vi "Post Process Noise Filter.vi"(0 "pInputImage":i32, 1 "iMode":i32, 2 "iHeight":i32, 5 "pOutputImage":i32, 7 "iOutputBufferSize":i32, 9 "iBaseline":i32, 11 "error in (no error)":errorcluster, 12 "fThreshold":sgl, 13 "iWidth":i32) -> (4 "pInputImage out":i32, 6 "pOutputImage out":i32, 8 "function return":u32, 15 "error out":errorcluster)   [LabVIEW 2014, in "atmcd32d.lvlib"]
doc: "unsigned int WINAPI PostProcessNoiseFilter(at_32 * pInputImage, at_32 * pOutputImage, int iOutputBufferSize, int iBaseline, int iMode, float fThreshold, int iHeight, int iWidth);"
uses:
  atmcd32d.lvlib
  atmcd32d.dll
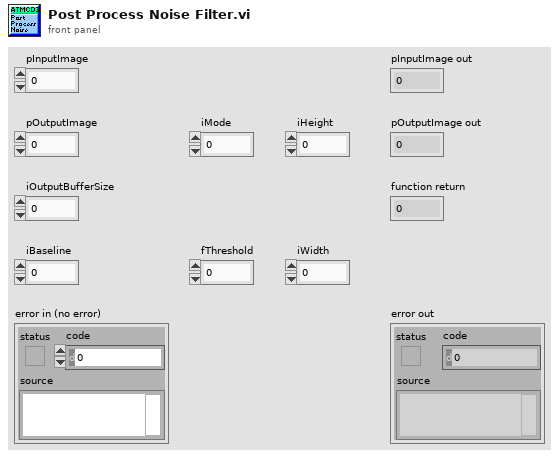
[diagram p1: front panel]
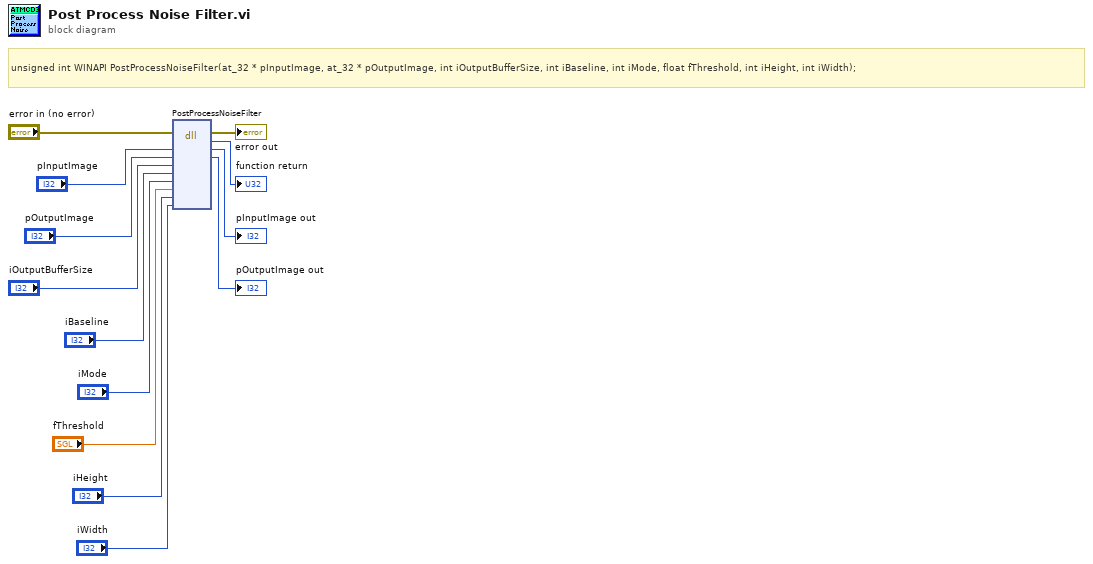
[diagram p0: block diagram]
diagram:
  # "unsigned int WINAPI PostProcessNoiseFilter(at_32 * pInputImage, at_32 * pOutputImage, int iOutputBufferSize, int iBaseline, int iMode, float fThreshold, int iHeight, int iWidth);"
  n1 = dll-call lib="C:/Users/Bakir/Documents/Lambda2-Testing/lib/Andorlib/atmcd32d.*" fn="PostProcessNoiseFilter"(error in="error in (no error)", "pInputImage"="pInputImage", "pOutputImage"="pOutputImage", "iOutputBufferSize"="iOutputBufferSize", "iBaseline"="iBaseline", "iMode"="iMode", "fThreshold"="fThreshold", "iHeight"="iHeight", "iWidth"="iWidth") -> (error out=→"error out":errorcluster, →"function return":u32, "pInputImage"=→"pInputImage out":i32, "pOutputImage"=→"pOutputImage out":i32)  [unwired: 8 in, 1 out]
